vi "sg Query Symbol Clock Rate.vi"(8 "error in (no error)":errorcluster, 10 "clock":dbl, 11 "device":i32) -> (0 "error out":errorcluster, 2 "clock out":dbl, 3 "function return":u32(ring))   [LabVIEW 2014, in "VSG25A.lvlib"]
doc: "SG_API sgStatus sgQuerySymbolClockRate(int device, double *clock);"
uses:
  VSG25A.lvlib
  sg_api.dll
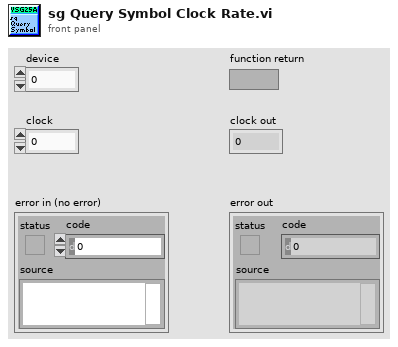
[diagram p1: front panel]
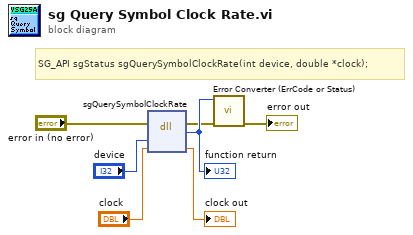
[diagram p0: block diagram]
diagram:
  # "SG_API sgStatus sgQuerySymbolClockRate(int device, double *clock);"
  n1 = dll-call lib="C:/Users/M_LAPTOP/Desktop/Labview/practice/VSG25A/sg_lib/sg_api.*" fn="sgQuerySymbolClockRate"(error in="error in (no error)", "device"="device", "clock"="clock") -> (error out=w2:errorcluster, w7:u32, "clock"=→"clock out":dbl)  [unwired: 3 in, 1 out]
  "function return" <- w7
  n2 = call "Error Converter (ErrCode or Status).vi"("error in (no error)"=w2, "error code"=w7) -> ("error out"=→"error out":errorcluster)  [unwired: 9 in]
